vi "get_header.vi"(8 "error in (no error)":errorcluster, 11 "ImageCollection in":refnum<class "ImageCollection.lvclass">) -> (0 "error out":errorcluster, 2 "header":refnum<class "XMLElement.lvclass">, 3 "ImageCollection out":refnum<class "ImageCollection.lvclass">)   [LabVIEW 2010, in "ImageCollection.lvclass"]
uses:
  ImageCollection.lvclass
  XMLElement/XMLElement/XMLElement.lvclass
  ImageCollection.lvclass/ImageCollection.ctl
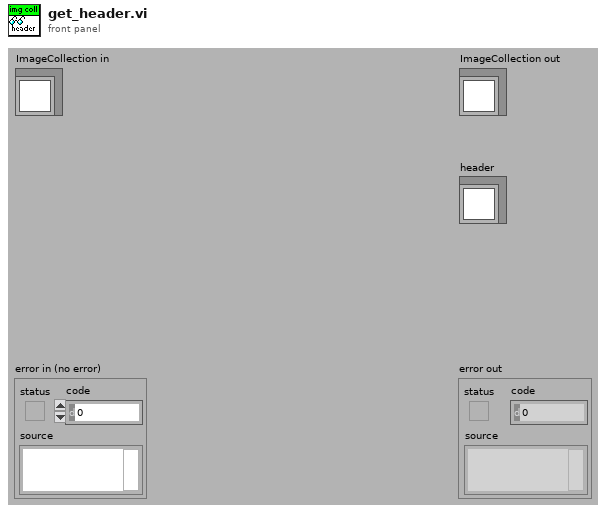
[diagram p1: front panel]
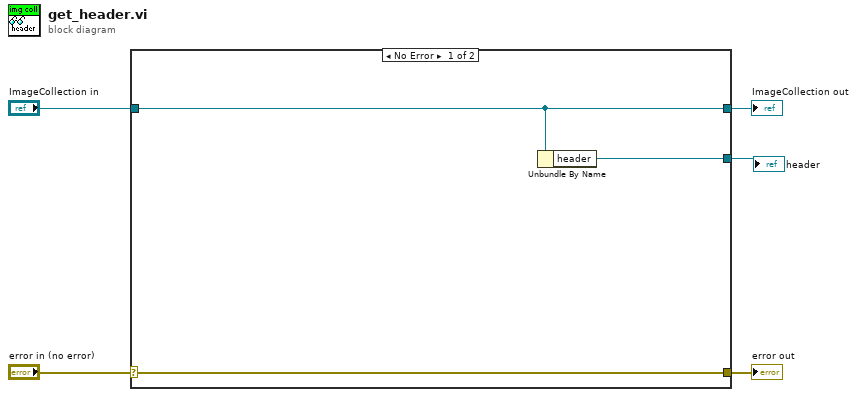
[diagram p0: block diagram]
diagram:
  n1 = case shown="No Error" "error in (no error)" {
    selector: "error in (no error)" -> [w8 w10]
    tunnel: [w8 w10] -> w4
    tunnel: [w7 w9] -> w2
    tunnel: "ImageCollection in" -> [w7 w9]
    tunnel: [w6 _] -> w1
    frame No Error {
      n2 = Unbundle By Name(w7) -> ("header"=w6:refnum<class "XMLElement.lvclass">)
    }
    frame Error {
    }
  }
  "error out" <- w4
  "ImageCollection out" <- w2
  "header" <- w1
